vi "Build SAEJ1850 CRC8 Table.vi"() -> (3 "CRC Table":u8[](array[numeric]))   [LabVIEW 2018, in "CAN Gateway Engine.lvlib"]
uses:
  CAN Gateway Engine.lvlib
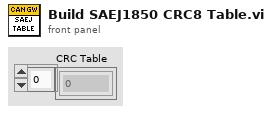
[diagram p1: front panel]
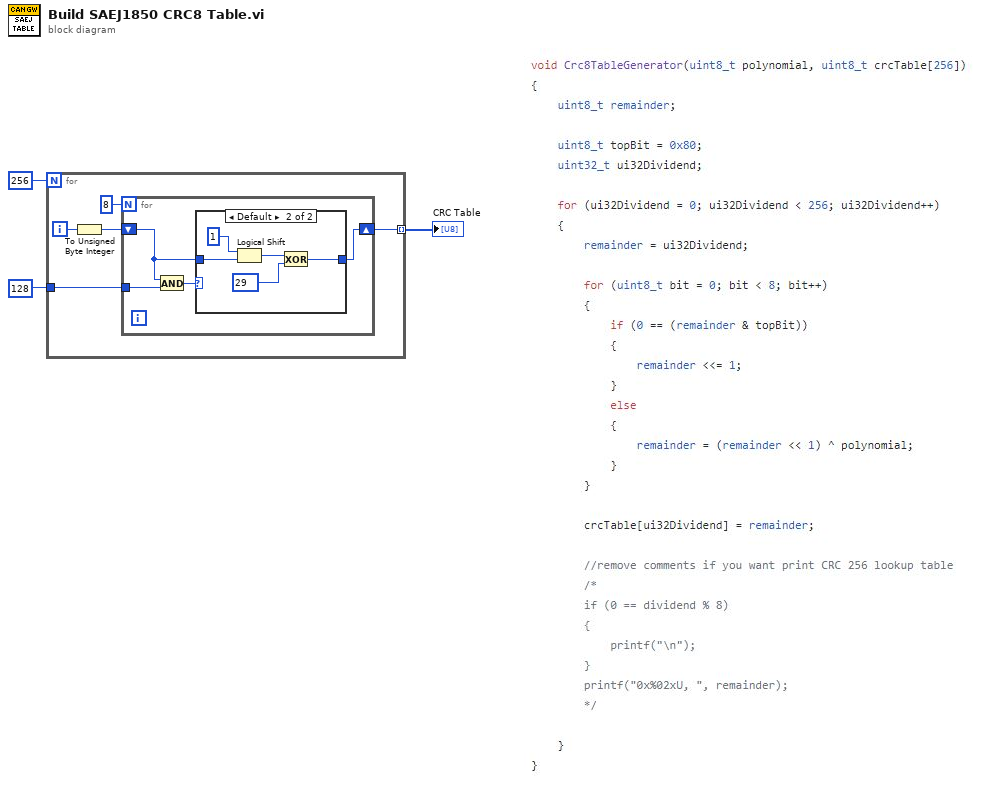
[diagram p0: block diagram]
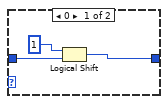
[diagram p2: hidden frame]
diagram:
  n1 = for {
    N: 256 -> [_]
    tunnel: u8 128 ("Numeric") -> [w8]
    tunnel: [w6] -> w3 mode=indexing
    i -> [w5]
    n2 = To Unsigned Byte Integer(number=w5) -> (unsigned 8bit integer=w4:u8)
    n3 = for {
      N: 8 -> [_]
      tunnel: w8 -> [w12]
      shift-right: [w9] -> w6
      shift-left: w4 -> [w10]
      n4 = And(x=w10, y=w12) -> (x .and. y?=w11:u8)
      n5 = case shown="Default" w11 {
        tunnel: w10 -> [w15 w19]
        tunnel: [w13 w17] -> w9
        frame 0 {
          n6 = Logical Shift(y=i16 1, x=w15) -> (x << y=w13:u8)
        }
        frame Default {
          n7 = Logical Shift(y=i16 1, x=w19) -> (x << y=w18:u8)
          n8 = Exclusive Or(1:u8 29 ("Numeric"), 2:w18) -> (0:w17:u8)
        }
      }
    }
  }
  "CRC Table" <- w3
